vi "VI Tree - time__ogtk.vi"   [LabVIEW 2018]
panel:
  # "[OpenG VI Tags] ***Do Not Remove***"
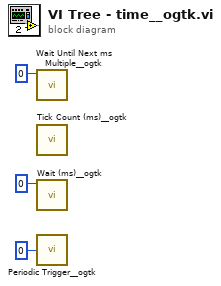
[diagram p0: block diagram]
diagram:
  n1 = call <userlib>:"Wait Until Next ms Multiple__ogtk.vi"("milliseconds to wait"=u32 0) -> ()  [unwired: 9 in, 2 out]
  n2 = call <userlib>:"Tick Count (ms)__ogtk.vi"() -> ()  [unwired: 10 in, 2 out]
  n3 = call <userlib>:"Wait (ms)__ogtk.vi"("milliseconds to wait"=u32 0) -> ()  [unwired: 9 in, 2 out]
  n4 = call <userlib>:"Periodic Trigger__ogtk.vi"("time (ms)"=u32 0) -> ()  [unwired: 12 in, 3 out]
